vi "Get String Contol Reference.vi"(11 "error in":errorcluster) -> (4 "string":refnum<vi>, 6 "vi reference":refnum<vi>, 15 "error out":errorcluster)   [LabVIEW 2021, in "Converter.lvlib"]
uses:
  Converter.lvlib
  Path Functions/Path Functions.lvlib
  Converter Reusables/Converter Reusables.lvlib
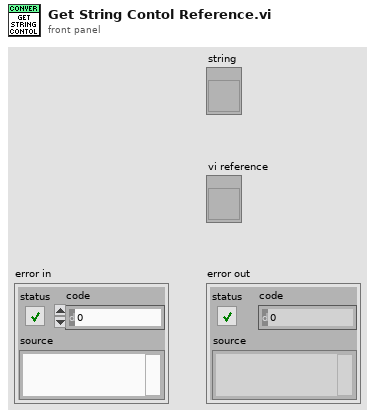
[diagram p1: front panel]
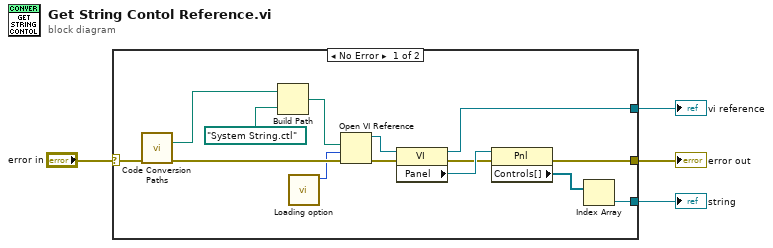
[diagram p0: block diagram]
diagram:
  n1 = case shown="No Error" "error in" {
    selector: "error in" -> [w8 w19]
    tunnel: [w9 _] -> w4
    tunnel: [w7 w19] -> w1
    tunnel: [w6 _] -> w2
    frame No Error {
      n2 = call "Code Conversion Paths.vi"("error in"=w8) -> ("io controls"=w17:path, "error out"=w13:errorcluster)  [unwired: 6 in, 7 out]
      n3 = Build Path(base path=w17, name or relative path=path "System String.ctl") -> (appended path=w16:path)
      n4 = call "Loading option.vi"() -> ("options"=w5:i32)  [unwired: 11 in]
      n5 = Open VI Reference(vi path=w16, options=w5, error in (no error)=w13) -> (vi reference=w10:refnum<vi>, error out=w12:errorcluster)  [unwired: 3 in]
      n6 = property class="VI"(reference=w10, error in=w12) -> (reference out=w6:refnum<vi>, error out=w11:errorcluster, "Panel"=w15:refnum<vi>)
      n7 = property class="Pnl"(reference=w15, error in=w11) -> (error out=w7:errorcluster, "Controls[]"=w14:refnum<vi>[])  [unwired: 1 out]
      n8 = Index Array(array=w14) -> (element=w9:refnum<vi>)  [unwired: 1 in]
    }
    frame Error {
    }
  }
  "string" <- w4
  "error out" <- w1
  "vi reference" <- w2
